vi "Fake Dust Events.vi"() -> ()   [LabVIEW 2009, in "Testing.lvlib"]
uses:
  Testing.lvlib
  interface/Dust Info.ctl
  interface/Timetrace.ctl
  interface/Data Source.ctl
  time/Time.lvlib
  interface/Interface.lvlib
panel:
  out "Iteration":i32
  in  "stop":bool
  out "error out":errorcluster
  in  "Array":T2(array[cluster])=[{"Source (CSA#, etc)"=enum."USER", "Data Role"=enum."USER", "Npoints"=10000.0}, {"Source (CSA#, etc)"=enum."CSA2", "Data Role"=enum."FIRST DETECTOR", "Npoints"=10000.0}, {"Source (CSA#, etc)"=enum."CSA3", "Data Role"=enum."SECOND DETECTOR", "Npoints"=10000.0}, {"Source (CSA#, etc)"=enum."CSA4", "Data Role"=enum."THIRD DETECTOR", "Npoints"=10000.0}, {"Source (CSA#, etc)"=enum."CSA6", "Data Role"=enum."FINAL DETECTOR", "Npoints"=10000.0}]
  in  "Rate (Hz)":dbl=1.0
  out "Out":T3
  in  "In":T3={"Time64"=0, "Velocity"=5000.0, "Charge"=5.0, "Mass"=11.0, "Time Traces"=[], "Selected"=FALSE}
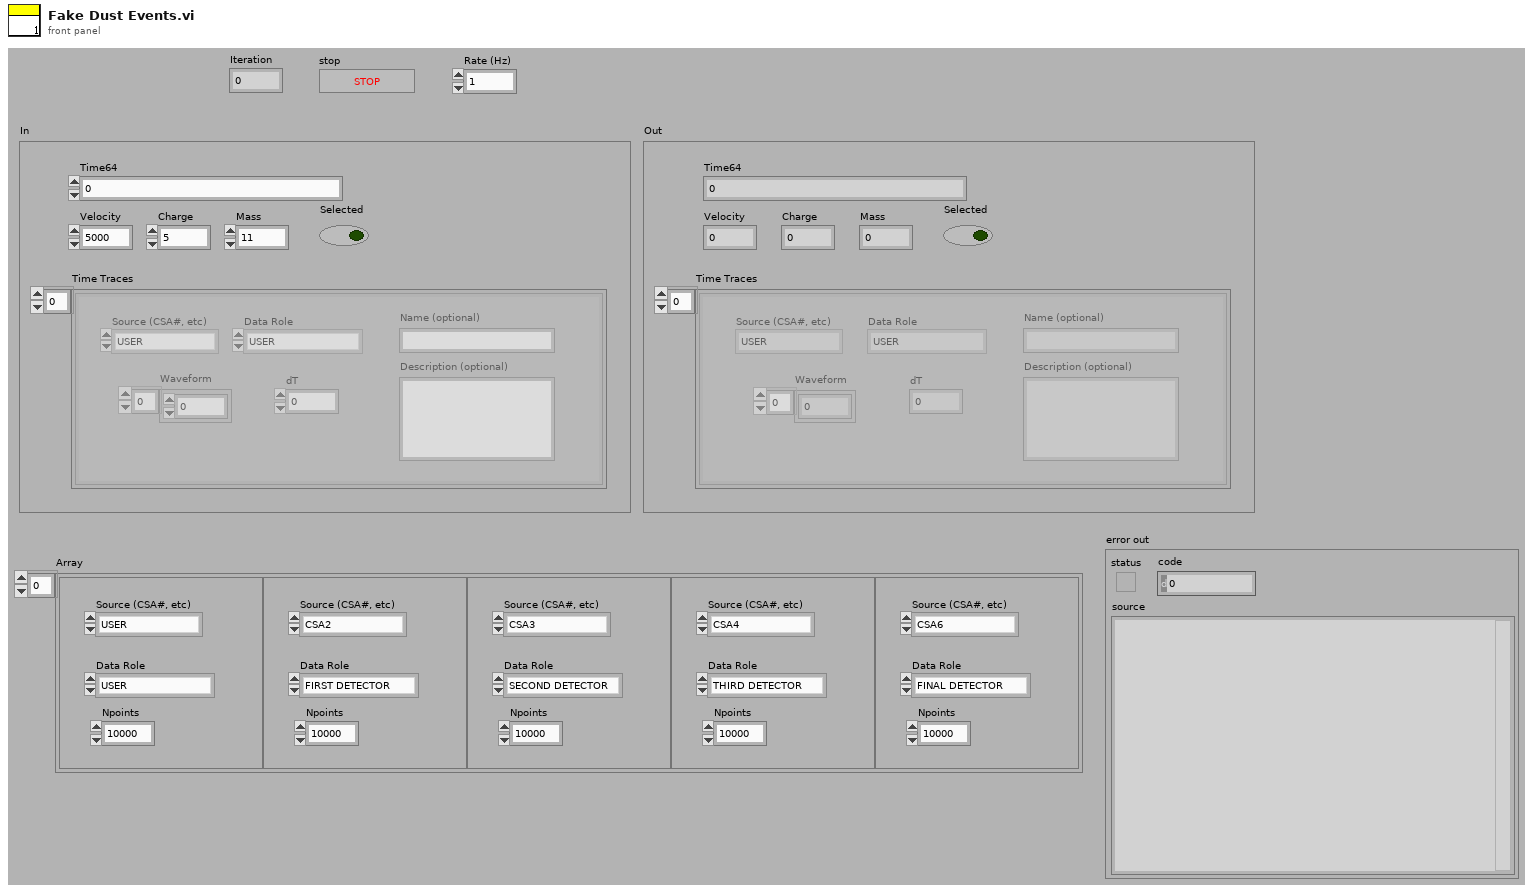
[diagram p1: front panel]
types:
  T1 = typedef "Interface.lvlib/Data Source.ctl" = enum16{"USER", "CSA1", "CSA2", "CSA3", "CSA4", "CSA5", "CSA6", ""}
  T2 = cluster{"Source (CSA#, etc)":T1, "Data Role":enum16{"USER", "FIRST DETECTOR", "SECOND DETECTOR", "THIRD DETECTOR", "FINAL DETECTOR"}, "Npoints":dbl}[]
  T3 = typedef "Interface.lvlib/Dust Info.ctl" = cluster{"Time64":u64, "Velocity":dbl, "Charge":dbl, "Mass":dbl, "Time Traces":T4[], "Selected":bool}
  T4 = typedef "Interface.lvlib/Timetrace.ctl" = cluster{"Source (CSA#, etc)":T1, "Data Role":enum16{"USER", "FIRST DETECTOR", "SECOND DETECTOR", "THIRD DETECTOR", "FINAL DETECTOR"}, "Waveform":sgl[], "dT":sgl, "Name (optional)":string, "Description (optional)":string}
  T5 = enum16{"USER", "FIRST DETECTOR", "SECOND DETECTOR", "THIRD DETECTOR", "FINAL DETECTOR"}
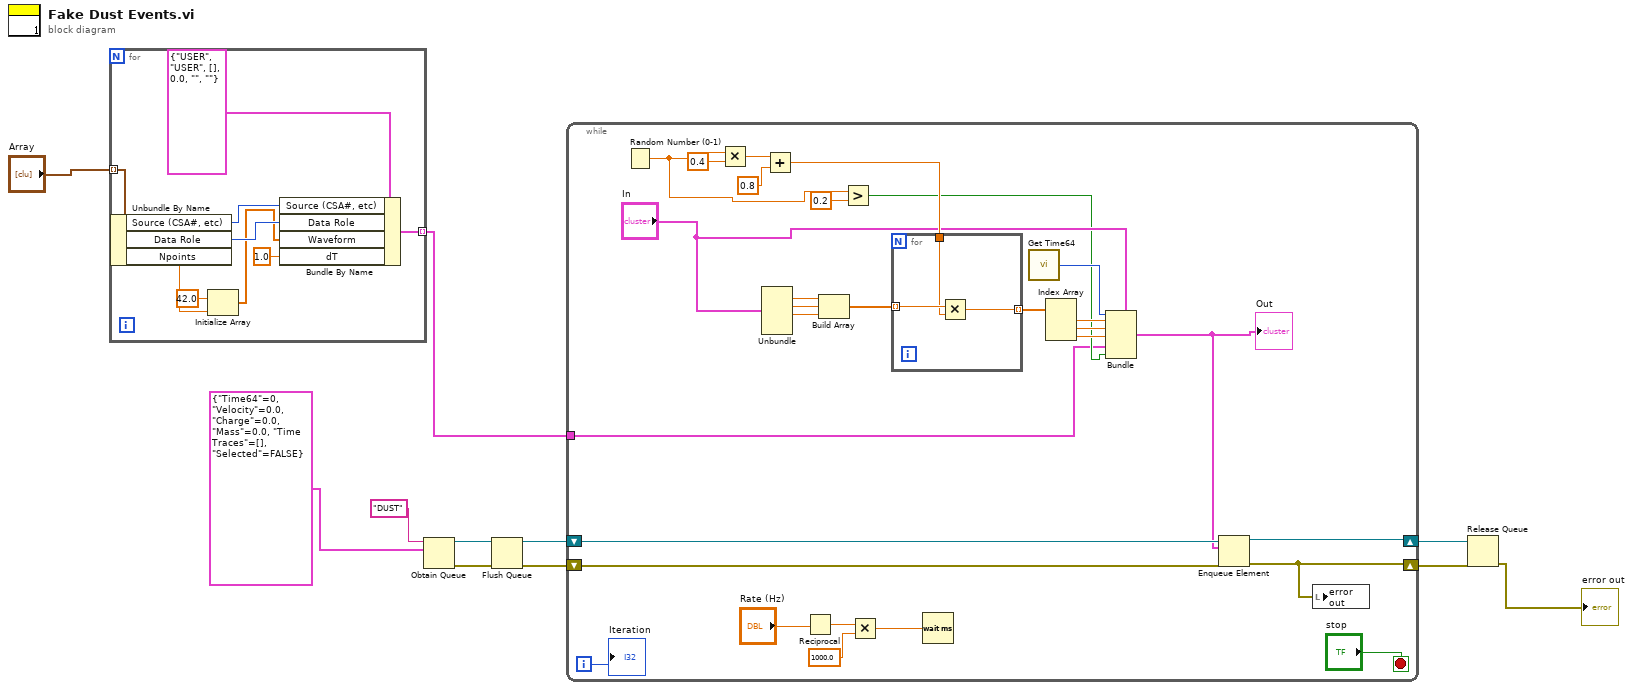
[diagram p0: block diagram]
diagram:
  n1 = for {
    tunnel: "Array" -> [w19] mode=indexing
    tunnel: [w12] -> w1 mode=indexing
    n2 = Unbundle By Name(w19) -> ("Source (CSA#, etc)"=w18:T1, "Data Role"=w17:T5, "Npoints"=w15:dbl)
    n3 = Initialize Array(42.0 ("element"), w15) -> (w13:dbl[])
    n4 = Bundle By Name(cluster=T4 {"Source (CSA#, etc)"=enum."USER", "Data Role"=enum."USER", "Waveform"=[], "dT"=0.0, "Name (optional)"="", "Description (optional)"=""} ("Cluster"), "Source (CSA#, etc)"=w18, "Data Role"=w17, "Waveform"=w13, "dT"=sgl 1.0) -> (w12:T4)
  }
  n5 = Obtain Queue(name (unnamed)="DUST", element data type=T3 {"Time64"=0, "Velocity"=0.0, "Charge"=0.0, "Mass"=0.0, "Time Traces"=[], "Selected"=FALSE} ("Cluster")) -> (queue out=w6:refnum<queue>, error out=w4:errorcluster)  [unwired: 3 in, 1 out]
  n6 = Flush Queue(queue=w6, error in (no error)=w4) -> (queue out=w5:refnum<queue>, error out=w3:errorcluster)  [unwired: 1 out]
  n7 = while {
    shift-right: [w30] -> w9
    shift-left: w5 -> [w32]
    shift-right: [w22] -> w8
    shift-left: w3 -> [w31]
    tunnel: w1 -> [w21]
    i -> [w28]
    stop <- "stop" stop-if-true
    n8 = Random Number (0-1)() -> (number: 0 to 1=w35:dbl)
    n9 = Multiply(x=w35, y=0.4) -> (x*y=w48:dbl)
    n10 = Unbundle("In") -> ("Velocity"=w46:dbl, "Charge"=w45:dbl, "Mass"=w44:dbl)  [unwired: 3 out]
    n11 = Add(x=w48, y=0.8) -> (x+y=w42:dbl)
    n12 = Reciprocal(x="Rate (Hz)") -> (1/x=w26:dbl)
    n13 = Build Array(w46, w45, w44) -> (w43:dbl[])
    n14 = Greater?(x=w35, y=0.2) -> (0:w33:bool)
    n15 = Multiply(x=w26, y=1000.0) -> (x*y=w24:dbl)
    n16 = for {
      tunnel: w43 -> [w52] mode=indexing
      tunnel: w42 -> [w51]
      tunnel: [w50] -> w39 mode=indexing
      n17 = Multiply(x=w52, y=w51) -> (x*y=w50:dbl)
    }
    n18 = Wait (ms)(milliseconds to wait=w24) -> ()  [unwired: 1 out]
    n19 = call "Get Time64.vi"() -> ("Labview time (ms)"=w40:u64)
    n20 = Index Array(array=w39) -> (element #1=w38:dbl, element #2=w37:dbl, element #3=w36:dbl)  [unwired: 3 in]
    n21 = Bundle(cluster="In", "Time64"=w40, "Velocity"=w38, "Charge"=w37, "Mass"=w36, "Time Traces"=w21, "Selected"=w33) -> (w23:T3)
    "Out" <- w23
    n22 = Enqueue Element(queue=w32, element=w23, error in (no error)=w31) -> (queue out=w30:refnum<queue>, error out=w22:errorcluster)  [unwired: 1 in, 1 out]
    n23 = local write "error out"(w22) -> ()
    "Iteration" <- w28
  }
  n24 = Release Queue(queue=w9, error in (no error)=w8) -> (error out=→"error out":errorcluster)  [unwired: 1 in, 2 out]
